vi "GGGGG.vi"() -> ()   [LabVIEW 2018]
panel:
  out "Boolean":bool
  # "GGGGGGG"
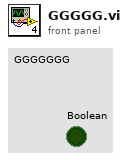
[diagram p1: front panel]
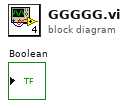
[diagram p0: block diagram]
diagram:
